vi "ExportMeasuresToPDF.vi"(8 "error in (no error)":errorcluster, 11 "Table in":refnum<vi>) -> (0 "error out":errorcluster)   [LabVIEW 2013]
uses:
  <userlib>/Exaprom PDF/Controls/Paragraphe cluster.ctl
  <userlib>/Exaprom PDF/Controls/Texte alignement.ctl
  <userlib>/Exaprom PDF/Controls/Line spacing.ctl
  <userlib>/Exaprom PDF/Controls/PDF Details.ctl
  <userlib>/Exaprom PDF/Controls/Image or Table Caption.ctl
  <userlib>/Exaprom PDF/Controls/Font cluster.ctl
  <userlib>/Exaprom PDF/Controls/Font size.ctl
  <userlib>/Exaprom PDF/Controls/Font color.ctl
  <userlib>/Exaprom PDF/Controls/Page setup.ctl
  <userlib>/Exaprom PDF/Controls/Page size.ctl
  <userlib>/Exaprom PDF/Controls/Page Orientation.ctl
  <userlib>/Exaprom PDF/Controls/Page Layout Custom.ctl
  <userlib>/Exaprom PDF/Controls/Page margins.ctl
  GlobalVariables/UserInfos.vi
  <userlib>/Exaprom PDF/VIs/Text/Append Paragraph.vi
  <userlib>/Exaprom PDF/VIs/Text/Append Phrase.vi
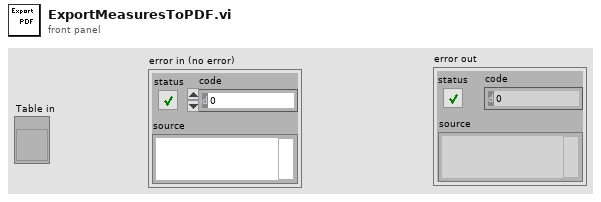
[diagram p1: front panel]
types:
  T1 = typedef "Font cluster.ctl" = cluster{"Name":string, "Size":T2, "Color":T3, "Style":cluster{"Bold":bool, "Italic":bool, "Underline":bool, "Strikeout":bool}}
  T2 = typedef "Font size.ctl" = sgl
  T3 = typedef "Font color.ctl" = u32
  T4 = typedef "Page setup.ctl" = cluster{"Page Size":T5, "Orientation":T6, "Custom Layout":T7, "Margins":T8}
  T5 = typedef "Page size.ctl" = i32
  T6 = typedef "Page Orientation.ctl" = enum16{"Portrait", "Landscape"}
  T7 = typedef "Page Layout Custom.ctl" = cluster{"Width":sgl, "Height":sgl}
  T8 = typedef "Page margins.ctl" = cluster{"Left":sgl, "Right":sgl, "Top":sgl, "Bottom":sgl}
  T9 = typedef "Paragraphe cluster.ctl" = cluster{" Aligment":T10, "Line spacing":T11}
  T10 = typedef "Texte alignement.ctl" = enum16{"Select", "CENTER", "JUSTIFY", "LEFT", "RIGHT"}
  T11 = typedef "Line spacing.ctl" = enum16{"Select", "1.0", "1.5", "2.0"}
  T12 = typedef "Image or Table Caption.ctl" = cluster{"Caption":string, "Separator":string, "Position":enum16{"Above", "Below"}}
  T13 = typedef "PDF Details.ctl" = cluster{"Title":string, "Subject":string, "Keywords":string, "Author":string, "Creator":string}
  T14 = cluster{"location":string, "Field":string, "Company":string, "Lab":string, "Operator":string, "Well":string, "Lat/Long":string, "Formation":string, "Country":string, "Client":string}
  T15 = typedef "Unit.ctl" = enum16{"inch", "mm"}
  T16 = typedef "Page dimensions.ctl" = cluster{"Start at page":i32, "Orientation":T6, "widht":sgl, "height":sgl, "Margin left":sgl, "Margin right":sgl, "Margin top":sgl, "Margin bottom":sgl}
  T17 = typedef "Header Footer [ ].ctl" = T18[]
  T18 = typedef "Header Footer cluster.ctl" = cluster{"Start page":i32, "Type":T19, "Alignment":T20, "Vertical Alignement":T21, "Image (%)":sgl, "Page #":T22, "Text":string, "Path":string, "Font":T1, "Font refnum":refnum<k24>, "Line":cluster{"Line":T23, "Thickness (points)":sgl, "Colour":T3}}
  T19 = typedef "Header Footer Type.ctl" = enum16{"Select", "Text", "Text + hyperlink", "Page number", "Image", "Image + hyperlink"}
  T20 = typedef "Header footer horiz alignment.ctl" = enum16{"Left", "Center", "Right"}
  T21 = typedef "Cell Vertical alignment.ctl" = enum16{"TOP", "MIDDLE", "BOTTOM"}
  T22 = typedef "Page number.ctl" = cluster{"Text 1":string, "Text 2":string, "Text 3":string}
  T23 = typedef "Header Footer Line.ctl" = enum16{"No line", "Horizontal line"}
  T24 = typedef "Watermark cluster2.ctl" = cluster{"Show? (F)":bool, "Type":enum16{"Image", "Text"}, "Opacity (%)":sgl, "Rotate(°)":sgl, "Position":cluster{"Position":T25, "X":sgl, "Y":sgl}, "Image path":path, "Scaled(%)":sgl, "Image refnum":refnum<k24>, "Text":string, "Font":cluster{"Name":string, "Size":T2, "Color":T3}, "Font refnum":refnum<k24>, "Alignment":T20, "Automatic":bool}
  T25 = typedef "Watermark Position.ctl" = enum16{"Absolute", "Center (page)", "Center (text section)"}
  T26 = typedef "System Fonts.ctl" = cluster{"Font name [ ]":string[], "Font and file names [ ]":cluster{"Font name":string, "File name":string}[]}
  T27 = cluster{"Document":refnum<k24>, "Writer":refnum<k24>, "Default Font":refnum<k24>, "Default Font cluster":T1, "Path":path, "Unit (default = mm)":T15, "Paragraphe cluster":T9, "Pages dimensions [ ]":T16[], "Captions":cluster{"Image":T12, "Image counter":u16, "Table":T12, "Table counter":u16, "Font":T1}, "Header":T17, "Footer":T17, "Watermark ":T24, "Actual VI name":string, "System Fonts":T26}
  T28 = cluster{"PDFTable ref":refnum<k24>, "columnWidth (points)":sgl[], "Title 1D":string[], "Table Datas 2D":string[][], "Image to Add with refnum[ ]":cluster{"Image name":string, "InstanceImage":refnum<k24>}[]}
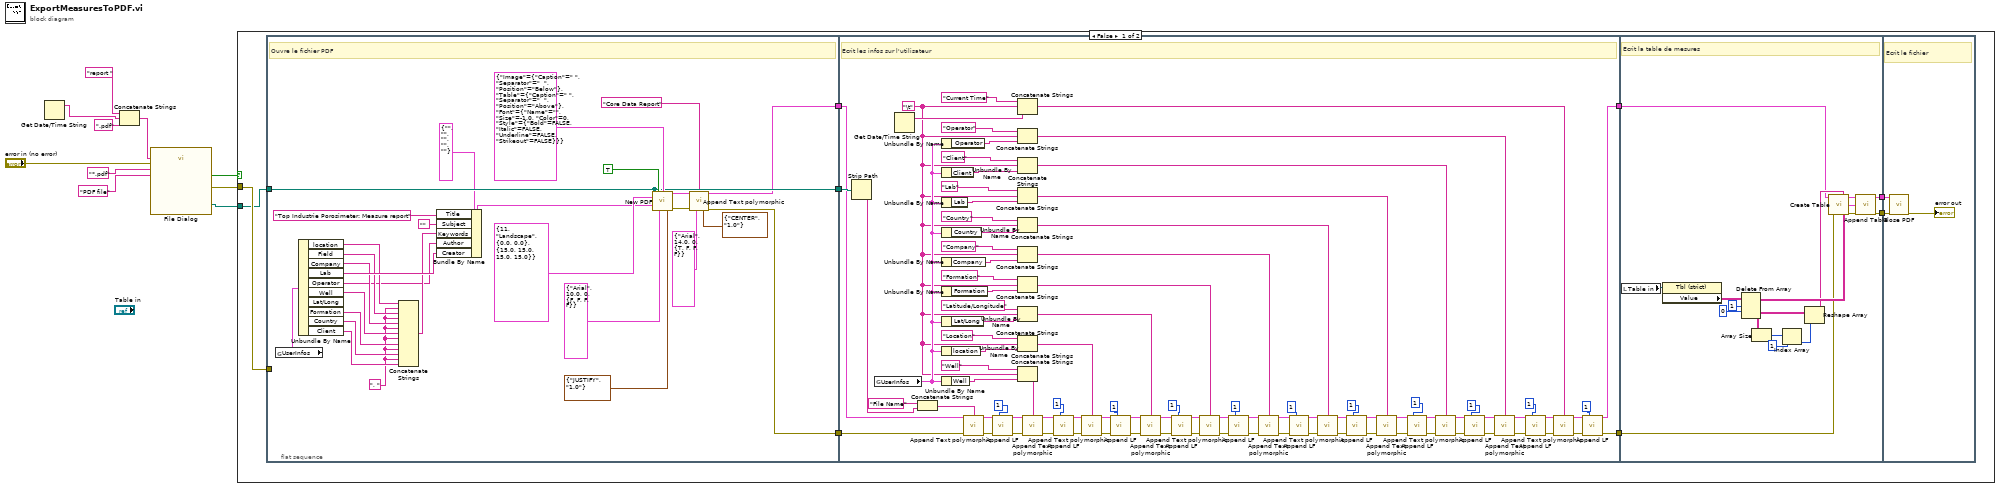
[diagram p0: block diagram]
diagram:
  n1 = Get Date/Time String() -> (date string=w2:string)  [unwired: 3 in, 1 out]
  n2 = Concatenate Strings("report " ("string"), w2, ".pdf" ("string")) -> (w3:string)
  n3 = call "File Dialog"("default name"=w3, "error in"="error in (no error)", "pattern (all files)"="*.pdf", "pattern label"="PDF file") -> ("selected path"=w6:path, "cancelled"=w1:bool, "error out"=w7:errorcluster)  [unwired: 8 in, 1 out]
  n4 = case shown="False" w1 {
    tunnel: w7 -> [w19 _]
    tunnel: w6 -> [w18 _]
    frame False {
      n5 = flat-sequence {
        tunnel: w19 -> [_]
        tunnel: w18 -> [w43]
        tunnel: [w43] -> w17
        tunnel: [w22] -> w16
        tunnel: [w23] -> w15
        tunnel: w17 -> [w141]
        tunnel: w16 -> [w107]
        tunnel: w15 -> [w62]
        tunnel: [w61] -> w14
        tunnel: [w60] -> w11
        tunnel: [w155] -> w13
        tunnel: w14 -> [w148]
        tunnel: [w146] -> w12
        tunnel: w11 -> [w147]
        tunnel: w13 -> [w160]
        tunnel: w12 -> [w159]
        frame #0 {
          w31 = ", "
          # "Ouvre le fichier PDF"
          n6 = global read "UserInfos.vi" "UserInfos"() -> (w42:T14)
          n7 = Unbundle By Name(w42) -> ("location"=w38:string, "Field"=w37:string, "Company"=w36:string, "Lab"=w41:string, "Operator"=w29:string, "Well"=w35:string, "Formation"=w34:string, "Country"=w33:string, "Client"=w32:string)  [unwired: 1 out]
          n8 = Concatenate Strings(w38, w31, w37, w31, w36, w31, w35, w31, w34, w31, w33, w31, w32) -> (w30:string)
          n9 = Bundle By Name(cluster=T13 {"Title"="", "Subject"="", "Keywords"="", "Author"="", "Creator"=""} ("PDF Details"), "Title"="Top Industrie Porosimeter: Measure report", "Subject"="", "Keywords"=w30, "Author"=w29, "Creator"=w41) -> (w39:T13)
          n10 = call <userlib>:"New PDF.vi"("PDF Path"=w43, "Overwrite?"=TRUE, "Captions"=cluster{"Image":T12, "Table":T12, "Font":T1} {"Image"={"Caption"=" ", "Separator"="  ", "Position"=enum."Below"}, "Table"={"Caption"=" ", "Separator"="  ", "Position"=enum."Above"}, "Font"={"Name"="", "Size"=-1.0, "Color"=0, "Style"={"Bold"=FALSE, "Italic"=FALSE, "Underline"=FALSE, "Strikeout"=FALSE}}}, "Page Setup"=T4 {"Page Size"=11, "Orientation"=enum."Landscape", "Custom Layout"={"Width"=0.0, "Height"=0.0}, "Margins"={"Left"=15.0, "Right"=15.0, "Top"=15.0, "Bottom"=15.0}}, "PDF Details"=w39, "Default Font"=T1 {"Name"="Arial", "Size"=10.0, "Color"=0, "Style"={"Bold"=FALSE, "Italic"=FALSE, "Underline"=FALSE, "Strikeout"=FALSE}}, "Default Paragraph"=T9 {" Aligment"=enum."JUSTIFY", "Line spacing"=enum."1.0"}) -> ("PDF Report"=w26:T27, "error out"=w25:errorcluster)  [unwired: 1 in, 6 out]
          n11 = call-poly <userlib>:"Append Text polymorphic.vi"("PDF Report"=w26, "Text"="Core Data Report", "error in (no error)"=w25, "Font"=T1 {"Name"="Arial", "Size"=14.0, "Color"=0, "Style"={"Bold"=TRUE, "Italic"=FALSE, "Underline"=FALSE, "Strikeout"=FALSE}}, "Paragraph properties"=T9 {" Aligment"=enum."CENTER", "Line spacing"=enum."1.0"}) -> ("PDF Report duplicate"=w22:T27, "error out"=w23:errorcluster)  [unwired: 9 in]
        }
        frame #1 {
          w49 = "\t"
          # "Ecrit les infos sur l'utilisateur"
          n12 = Strip Path(path=w141) -> (name=w109:string)  [unwired: 1 out]
          n13 = global read "UserInfos.vi" "UserInfos"() -> (w85:T14)
          n14 = Get Date/Time String() -> (date string=w50:string)  [unwired: 3 in, 1 out]
          n15 = Concatenate Strings("File Name", w109) -> (w108:string)
          n16 = Unbundle By Name(w85) -> ("Operator"=w51:string)
          n17 = Unbundle By Name(w85) -> ("Client"=w52:string)
          n18 = Unbundle By Name(w85) -> ("Lab"=w53:string)
          n19 = Unbundle By Name(w85) -> ("Country"=w54:string)
          n20 = Unbundle By Name(w85) -> ("Company"=w55:string)
          n21 = Unbundle By Name(w85) -> ("Formation"=w56:string)
          n22 = Unbundle By Name(w85) -> ("Lat/Long"=w57:string)
          n23 = Unbundle By Name(w85) -> ("location"=w58:string)
          n24 = Unbundle By Name(w85) -> ("Well"=w59:string)
          n25 = call-poly <userlib>:"Append Text polymorphic.vi"("PDF Report IN"=w107, "Text"=w108, "error in (no error)"=w62) -> ("PDF Report OUT"=w140:T27, "error out"=w139:errorcluster)  [unwired: 11 in]
          n26 = call <userlib>:"Append LF.vi"("PDF Report IN"=w140, "Number of LF (default 1)"=1, "error in (no error)"=w139) -> ("PDF Report duplicate"=w138:T27, "error out"=w137:errorcluster)  [unwired: 11 in]
          n27 = Concatenate Strings("Current Time", w49, w50) -> (w63:string)
          n28 = Concatenate Strings("Operator", w49, w51) -> (w65:string)
          n29 = Concatenate Strings("Client", w49, w52) -> (w66:string)
          n30 = Concatenate Strings("Lab", w49, w53) -> (w82:string)
          n31 = Concatenate Strings("Country", w49, w54) -> (w83:string)
          n32 = Concatenate Strings("Company", w49, w55) -> (w84:string)
          n33 = Concatenate Strings("Formation", w49, w56) -> (w91:string)
          n34 = Concatenate Strings("Latitude/Longitude", w49, w57) -> (w93:string)
          n35 = Concatenate Strings("Location", w49, w58) -> (w95:string)
          n36 = Concatenate Strings("Well", w49, w59) -> (w97:string)
          n37 = call-poly <userlib>:"Append Text polymorphic.vi"("PDF Report IN"=w138, "Text"=w97, "error in (no error)"=w137) -> ("PDF Report OUT"=w136:T27, "error out"=w135:errorcluster)  [unwired: 11 in]
          n38 = call <userlib>:"Append LF.vi"("PDF Report IN"=w136, "Number of LF (default 1)"=1, "error in (no error)"=w135) -> ("PDF Report duplicate"=w127:T27, "error out"=w128:errorcluster)  [unwired: 11 in]
          n39 = call-poly <userlib>:"Append Text polymorphic.vi"("PDF Report IN"=w127, "Text"=w95, "error in (no error)"=w128) -> ("PDF Report OUT"=w134:T27, "error out"=w133:errorcluster)  [unwired: 11 in]
          n40 = call <userlib>:"Append LF.vi"("PDF Report IN"=w134, "Number of LF (default 1)"=1, "error in (no error)"=w133) -> ("PDF Report duplicate"=w132:T27, "error out"=w131:errorcluster)  [unwired: 11 in]
          n41 = call-poly <userlib>:"Append Text polymorphic.vi"("PDF Report IN"=w132, "Text"=w93, "error in (no error)"=w131) -> ("PDF Report OUT"=w130:T27, "error out"=w129:errorcluster)  [unwired: 11 in]
          n42 = call <userlib>:"Append LF.vi"("PDF Report IN"=w130, "Number of LF (default 1)"=1, "error in (no error)"=w129) -> ("PDF Report duplicate"=w111:T27, "error out"=w112:errorcluster)  [unwired: 11 in]
          n43 = call-poly <userlib>:"Append Text polymorphic.vi"("PDF Report IN"=w111, "Text"=w91, "error in (no error)"=w112) -> ("PDF Report OUT"=w126:T27, "error out"=w125:errorcluster)  [unwired: 11 in]
          n44 = call <userlib>:"Append LF.vi"("PDF Report IN"=w126, "Number of LF (default 1)"=1, "error in (no error)"=w125) -> ("PDF Report duplicate"=w124:T27, "error out"=w123:errorcluster)  [unwired: 11 in]
          n45 = call-poly <userlib>:"Append Text polymorphic.vi"("PDF Report IN"=w124, "Text"=w84, "error in (no error)"=w123) -> ("PDF Report OUT"=w122:T27, "error out"=w121:errorcluster)  [unwired: 11 in]
          n46 = call <userlib>:"Append LF.vi"("PDF Report IN"=w122, "Number of LF (default 1)"=1, "error in (no error)"=w121) -> ("PDF Report duplicate"=w113:T27, "error out"=w114:errorcluster)  [unwired: 11 in]
          n47 = call-poly <userlib>:"Append Text polymorphic.vi"("PDF Report IN"=w113, "Text"=w83, "error in (no error)"=w114) -> ("PDF Report OUT"=w120:T27, "error out"=w119:errorcluster)  [unwired: 11 in]
          n48 = call <userlib>:"Append LF.vi"("PDF Report IN"=w120, "Number of LF (default 1)"=1, "error in (no error)"=w119) -> ("PDF Report duplicate"=w118:T27, "error out"=w117:errorcluster)  [unwired: 11 in]
          n49 = call-poly <userlib>:"Append Text polymorphic.vi"("PDF Report IN"=w118, "Text"=w82, "error in (no error)"=w117) -> ("PDF Report OUT"=w116:T27, "error out"=w115:errorcluster)  [unwired: 11 in]
          n50 = call <userlib>:"Append LF.vi"("PDF Report IN"=w116, "Number of LF (default 1)"=1, "error in (no error)"=w115) -> ("PDF Report duplicate"=w68:T27, "error out"=w67:errorcluster)  [unwired: 11 in]
          n51 = call-poly <userlib>:"Append Text polymorphic.vi"("PDF Report IN"=w68, "Text"=w66, "error in (no error)"=w67) -> ("PDF Report OUT"=w81:T27, "error out"=w80:errorcluster)  [unwired: 11 in]
          n52 = call <userlib>:"Append LF.vi"("PDF Report IN"=w81, "Number of LF (default 1)"=1, "error in (no error)"=w80) -> ("PDF Report duplicate"=w79:T27, "error out"=w78:errorcluster)  [unwired: 11 in]
          n53 = call-poly <userlib>:"Append Text polymorphic.vi"("PDF Report IN"=w79, "Text"=w65, "error in (no error)"=w78) -> ("PDF Report OUT"=w77:T27, "error out"=w76:errorcluster)  [unwired: 11 in]
          n54 = call <userlib>:"Append LF.vi"("PDF Report IN"=w77, "Number of LF (default 1)"=1, "error in (no error)"=w76) -> ("PDF Report duplicate"=w72:T27, "error out"=w73:errorcluster)  [unwired: 11 in]
          n55 = call-poly <userlib>:"Append Text polymorphic.vi"("PDF Report IN"=w72, "Text"=w63, "error in (no error)"=w73) -> ("PDF Report OUT"=w75:T27, "error out"=w74:errorcluster)  [unwired: 11 in]
          n56 = call <userlib>:"Append LF.vi"("PDF Report IN"=w75, "Number of LF (default 1)"=1, "error in (no error)"=w74) -> ("PDF Report duplicate"=w61:T27, "error out"=w60:errorcluster)  [unwired: 11 in]
        }
        frame #2 {
          # "Ecrit la table de mesures"
          n57 = local read "Table in"() -> (w154:refnum<vi>)
          n58 = property on="Property Node" class="Tbl (strict)"(reference=w154) -> ("Value"=w153:string[][])  [unwired: 1 in, 2 out]
          n59 = Delete From Array(array=w153, length=1, index (row)=0) -> (deleted portion=w145:string[][], array with subset deleted=w150:string[][])  [unwired: 1 in]
          n60 = Array Size(array=w145) -> (size(s)=w144:i32[])
          n61 = Index Array(array=w144, index=1) -> (element=w142:i32)
          n62 = Reshape Array(w145, w142) -> (w149:string[])
          n63 = call <userlib>:"Create Table.vi"("PDF Report"=w148, "Title 1D"=w149, "error in (no error)"=w147, "Table Datas 2D"=w150) -> ("PDF Report duplicate"=w158:T27, "PDF Table"=w157:T28, "error out"=w156:errorcluster)  [unwired: 9 in]
          n64 = call <userlib>:"Append Table.vi"("PDF Report IN"=w158, "PDF Table"=w157, "error in (no error)"=w156) -> ("PDF Report OUT"=w155:T27, "error out"=w146:errorcluster)  [unwired: 11 in]
        }
        frame #3 {
          # "Ecrit le fichier"
          n65 = call <userlib>:"Close PDF.vi"("PDF Report"=w160, "error in (no error)"=w159) -> ("error out"=→"error out":errorcluster)  [unwired: 12 in, 1 out]
        }
      }
    }
    frame True {
    }
  }
